vi "soglia.vi"(5 "valore di controllo":dbl=4.0, 7 "index":i32=2, 11 "waveform_in":waveform(dbl)[](array[waveform])) -> (2 "waveform_out_single":waveform(dbl), 3 "Boolean":bool)   [LabVIEW 2017]
uses:
  <vilib>/Waveform/WDTOps.llb/WDT Index Channel DBL.vi
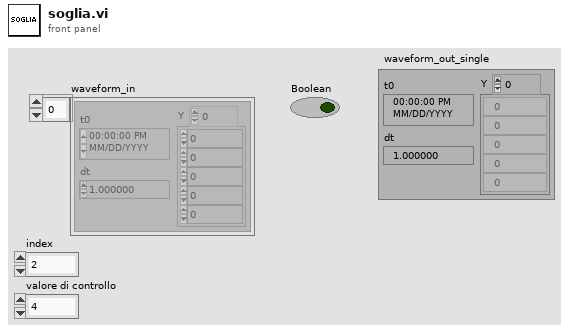
[diagram p1: front panel]
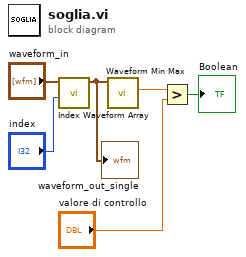
[diagram p0: block diagram]
diagram:
  n1 = call-poly <vilib>:"Index Waveform Array.vi"("index"="index", "waveform array"="waveform_in") -> ("waveform"=w4:waveform(dbl))  [unwired: 8 in, 1 out]
  "waveform_out_single" <- w4
  n2 = call <vilib>:"Waveform Min Max.vi"("waveform in"=w4) -> ("Y max"=w5:dbl)  [unwired: 5 in, 5 out]
  n3 = Greater?(x=w5, y="valore di controllo") -> (0:→"Boolean":bool)
